vi "1kW_SubVI.vi"() -> ()   [LabVIEW 2020]
panel:
  out "Step 4\nIndicator":bool
  out "Step 6\nIndicator":bool
  out "Step 5\nIndicator":bool
  out "Step 3\nIndicator":bool
  out "Step 2\nIndicator":bool
  out "Step 1\nIndicator":bool
  in  "Stop":bool
  out "Voltage (V)":dbl
  in  "Power Supply":bool
  out "B":bool
  out "Y":bool
  out "R":bool
  out "No. of Resistors Used":i32
  in  "Step Type":enum32{"Variable Steps", "Equal Steps"}(tab)
  in  "Step 1\n50W":bool
  in  "Step 2\n100W":bool
  in  "Step 3\n150W":bool
  in  "Step 4\n200W":bool
  in  "Step 5\n250W":bool
  in  "Step 6\n250W":bool
  in  "No. of Equal Steps":enum32{"2 Steps", "4 Steps"}(tab)
  in  "Step 2\n500W":bool
  in  "Step 1\n500W":bool
  in  "Step 4\n250W":bool
  in  "Step 3\n250W":bool
  in  "Step 2\n250W":bool
  in  "Step 1\n250W":bool
  in  "Master Switch":bool
  out "Load (kW)":dbl
  out "Current (A)":dbl format="%.4f"
  # "Three Phase Variable Resistive Load Bank with 1kW Maximum Capacity and 6 Step Control"
  # "All resistors are connected in 3 phase star formation"
  # "3 Phase Voltage Indicator"
  # "Each Resistor Looks Like This"
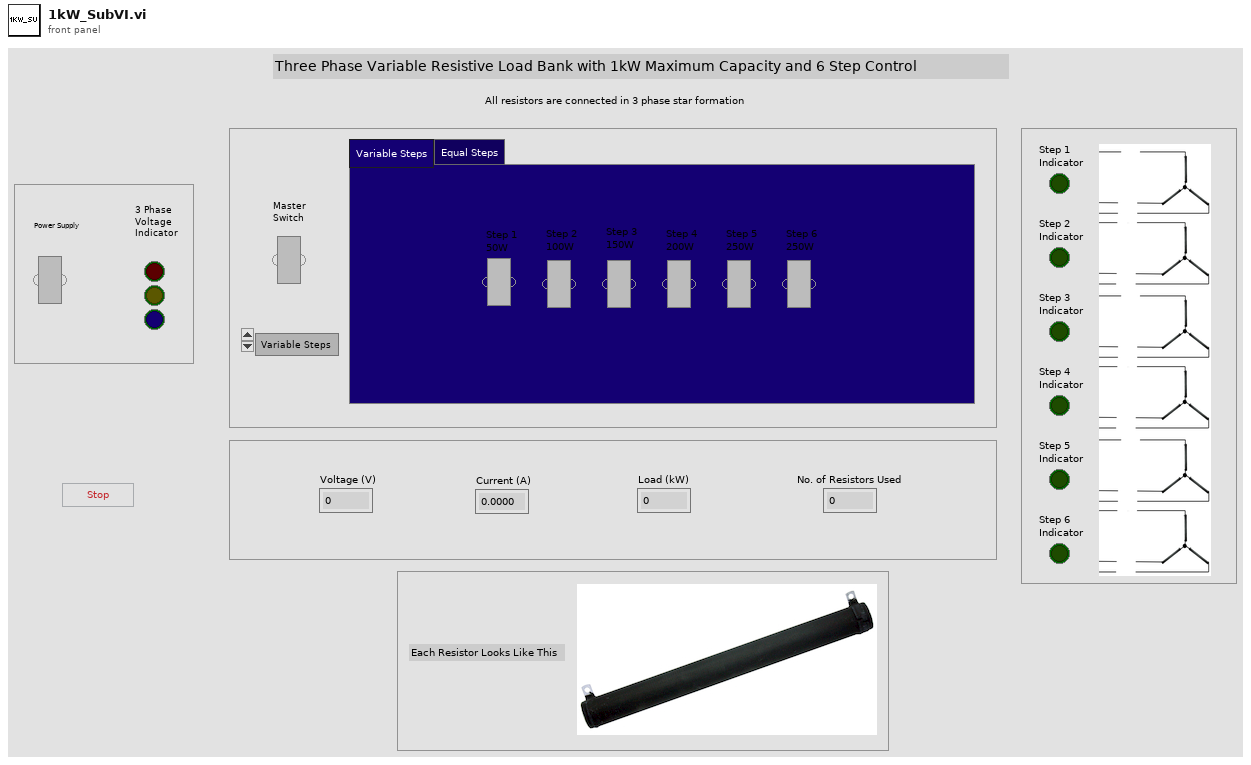
[diagram p1: front panel]
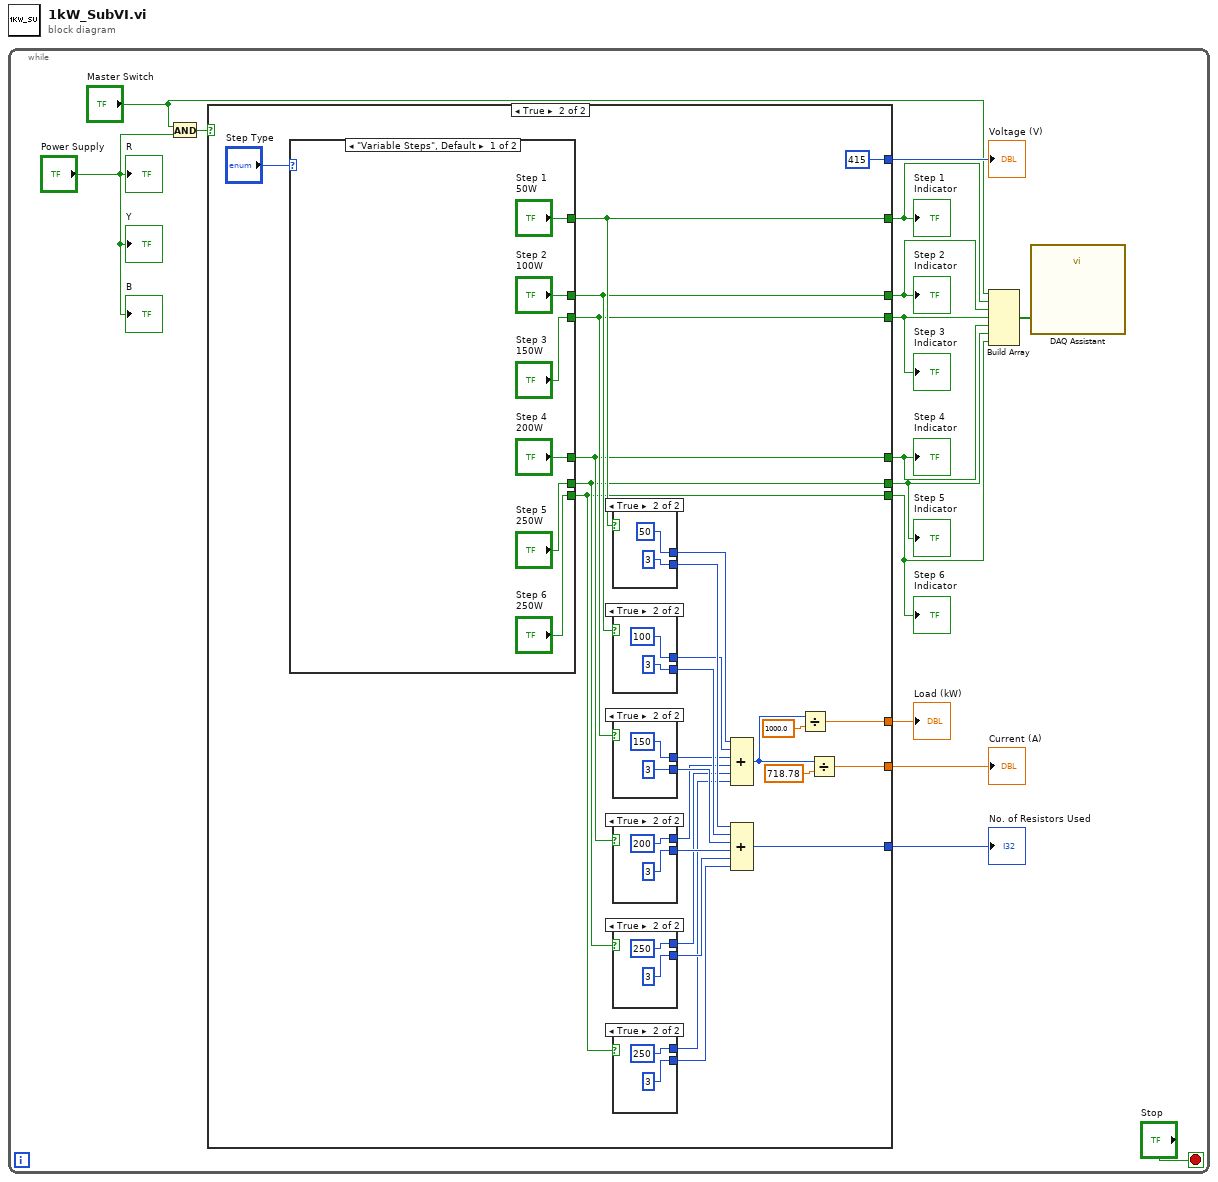
[diagram p0: block diagram]
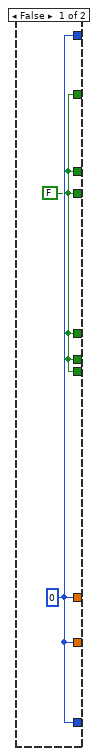
[diagram p2: hidden frame]
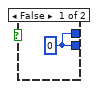
[diagram p3: hidden frame]
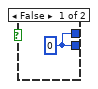
[diagram p4: hidden frame]
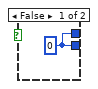
[diagram p5: hidden frame]
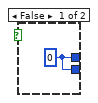
[diagram p6: hidden frame]
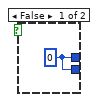
[diagram p7: hidden frame]
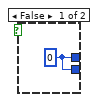
[diagram p8: hidden frame]
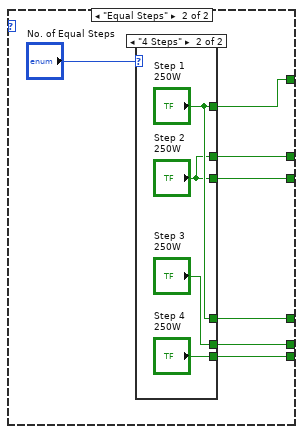
[diagram p9: hidden frame]
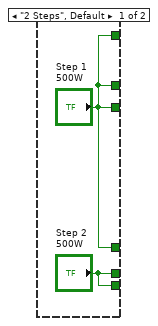
[diagram p10: hidden frame]
diagram:
  n1 = while {
    stop <- "Stop" stop-if-true
    n2 = And(x="Master Switch", y="Power Supply") -> (x .and. y?=w11:bool)
    n3 = case shown="True" w11 {
      tunnel: [w17 w28] -> w14
      tunnel: [w17 w24] -> w13
      tunnel: [w17 w25] -> w15
      tunnel: [w17 415] -> w12
      tunnel: [w16 w23] -> w3
      tunnel: [w16 w22] -> w4
      tunnel: [w16 w21] -> w5
      tunnel: [w16 w20] -> w6
      tunnel: [w16 w19] -> w2
      tunnel: [w16 w18] -> w1
      frame False {
        w16 = FALSE
        w17 = 0
      }
      frame True {
        n4 = case shown="\"Variable Steps\", Default" "Step Type" {
          tunnel: ["Step 6\n250W" w69] -> w18
          tunnel: ["Step 5\n250W" w70] -> w19
          tunnel: ["Step 4\n200W" w71] -> w20
          tunnel: ["Step 3\n150W" w72] -> w21
          tunnel: ["Step 2\n100W" w73] -> w22
          tunnel: ["Step 1\n50W" w74] -> w23
          frame "Variable Steps", Default {
          }
          frame "Equal Steps" {
            n5 = case shown="\"4 Steps\"" "No. of Equal Steps" {
              tunnel: ["Step 1\n500W" "Step 1\n250W"] -> w74
              tunnel: ["Step 1\n500W" "Step 2\n250W"] -> w73
              tunnel: ["Step 1\n500W" "Step 2\n250W"] -> w72
              tunnel: ["Step 1\n500W" "Step 1\n250W"] -> w71
              tunnel: ["Step 2\n500W" "Step 3\n250W"] -> w70
              tunnel: ["Step 2\n500W" "Step 4\n250W"] -> w69
              frame "2 Steps", Default {
              }
              frame "4 Steps" {
              }
            }
          }
        }
        n6 = case shown="True" w23 {
          tunnel: [w59 50] -> w29
          tunnel: [w59 3] -> w35
          frame False {
            w59 = 0
          }
          frame True {
          }
        }
        n7 = case shown="True" w22 {
          tunnel: [w56 100] -> w30
          tunnel: [w56 3] -> w36
          frame False {
            w56 = 0
          }
          frame True {
          }
        }
        n8 = case shown="True" w21 {
          tunnel: [w53 150] -> w31
          tunnel: [w53 3] -> w37
          frame False {
            w53 = 0
          }
          frame True {
          }
        }
        n9 = case shown="True" w20 {
          tunnel: [w50 200] -> w32
          tunnel: [w50 3] -> w38
          frame False {
            w50 = 0
          }
          frame True {
          }
        }
        n10 = case shown="True" w19 {
          tunnel: [w47 250] -> w33
          tunnel: [w47 3] -> w39
          frame False {
            w47 = 0
          }
          frame True {
          }
        }
        n11 = case shown="True" w18 {
          tunnel: [w44 250] -> w34
          tunnel: [w44 3] -> w40
          frame False {
            w44 = 0
          }
          frame True {
          }
        }
        n12 = Compound Arithmetic op=ADD(w29, w30, w31, w32, w33, w34) -> (w27:i32)
        n13 = Compound Arithmetic op=ADD(w35, w36, w37, w38, w39, w40) -> (w28:i32)
        n14 = Divide(x=w27, y=1000.0) -> (x/y=w25:dbl)
        n15 = Divide(x=w27, y=718.78) -> (x/y=w24:dbl)
      }
    }
    "Load (kW)" <- w15
    "Current (A)" <- w13
    "No. of Resistors Used" <- w14
    "Voltage (V)" <- w12
    "Step 1\nIndicator" <- w3
    "Step 2\nIndicator" <- w4
    "Step 3\nIndicator" <- w5
    "Step 4\nIndicator" <- w6
    "Step 5\nIndicator" <- w2
    "Step 6\nIndicator" <- w1
    n16 = Build Array("Master Switch", w3, w4, w5, w6, w2, w1) -> (w9:bool[])
    n17 = call "DAQ Assistant"("data"=w9) -> ()  [unwired: 17 in, 2 out]
    "B" <- "Power Supply"
    "Y" <- "Power Supply"
    "R" <- "Power Supply"
  }
